vi "Rinocloud_local_mirror.vi"(8 "error in":errorcluster, 9 "JSON payload":string, 10 "file name":string, 11 "file path":path) -> (0 "error out":errorcluster)   [LabVIEW 2013, in "Rinocloud Library.lvlib"]
uses:
  Rinocloud Library.lvlib
  Rinocloud_global_variable.vi
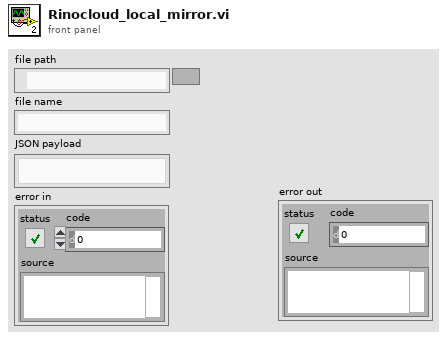
[diagram p1: front panel]
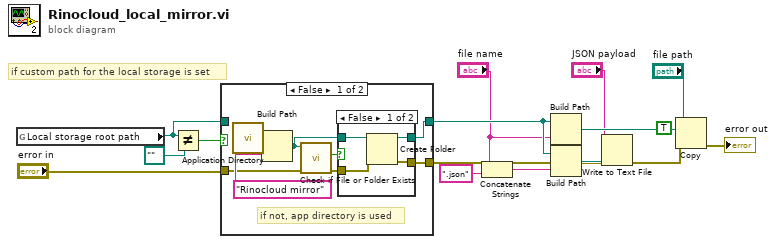
[diagram p0: block diagram]
diagram:
  # "if custom path for the local storage is set"
  n1 = global read "Rinocloud_global_variable.vi" "Local storage root path"() -> (w9:path)
  n2 = Not Equal?(x=w9, y=path "") -> (x != y?=w10:bool)
  n3 = case shown="False" w10 {
    tunnel: w9 -> [_ w32]
    tunnel: [w19 w32] -> w8
    tunnel: [w18 w31] -> w7
    tunnel: "error in" -> [w17 w31]
    frame False {
      # "if not, app directory is used"
      n4 = call <vilib>:"Application Directory.vi"() -> ("Application Directory"=w20:path)
      n5 = Build Path(base path=w20, name or relative path="Rinocloud mirror") -> (appended path=w23:path)
      n6 = call <vilib>:"Check if File or Folder Exists.vi"("error in (no error)"=w17, "path"=w23) -> ("error out"=w24:errorcluster, "file or folder exists?"=w22:bool)  [unwired: 7 in, 1 out]
      n7 = case shown="False" w22 {
        tunnel: [w25 w30] -> w19
        tunnel: w23 -> [w28 w30]
        tunnel: w24 -> [w27 w29]
        tunnel: [w26 w29] -> w18
        frame False {
          n8 = Create Folder(path (use dialog)=w28, error in=w27) -> (created path=w25:path, error out=w26:errorcluster)  [unwired: 1 in, 1 out]
        }
        frame True {
        }
      }
    }
    frame True {
    }
  }
  n9 = Concatenate Strings("file name", ".json" ("string")) -> (w13:string)
  n10 = Build Path(base path=w8, name or relative path="file name") -> (appended path=w15:path)
  n11 = Build Path(base path=w8, name or relative path=w13) -> (appended path=w12:path)
  n12 = Write to Text File(file (use dialog)=w12, text="JSON payload", error in=w7) -> (error out=w11:errorcluster)  [unwired: 1 in, 2 out]
  n13 = Copy(8:w11, 9:TRUE ("overwrite (F)"), 10:w15, 11:"file path") -> (0:→"error out":errorcluster)  [unwired: 1 in, 2 out]
